vi "store constructor.vi"(11 "Store type":T1(array[ring])=[enum."AD_STORE_DISCRETE"]) -> (3 "Store ID":i32)   [LabVIEW 2021, in "libad4.lvlib"]
doc: "Helper to make setting the store type easier."
uses:
  <userlib>/libad4/libad4.lvlib
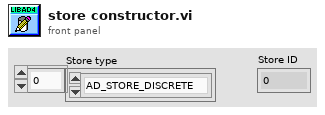
[diagram p1: front panel]
types:
  T1 = enum16{"AD_STORE_DISCRETE", "AD_STORE_AVERAGE", "AD_STORE_MIN", "AD_STORE_MAX", "AD_STORE_RMS"}[]
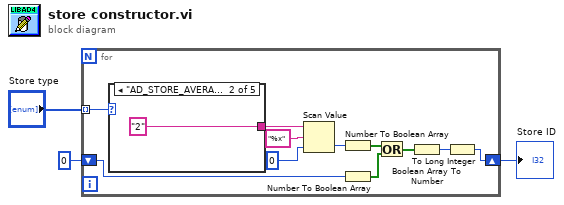
[diagram p0: block diagram]
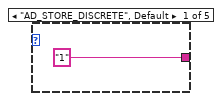
[diagram p2: hidden frame]
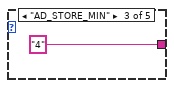
[diagram p3: hidden frame]
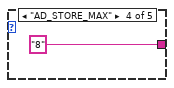
[diagram p4: hidden frame]
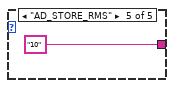
[diagram p5: hidden frame]
diagram:
  n1 = for {
    tunnel: "Store type" -> [w12] mode=indexing
    shift-right: [w6] -> w3
    shift-left: 0 -> [w5]
    n2 = case shown="\"AD_STORE_AVERAGE\"" w12 {
      tunnel: ["1" "2" "4" "8" "10"] -> w13
      frame "AD_STORE_DISCRETE", Default {
      }
      frame "AD_STORE_AVERAGE" {
      }
      frame "AD_STORE_MIN" {
      }
      frame "AD_STORE_MAX" {
      }
      frame "AD_STORE_RMS" {
      }
    }
    n3 = Scan Value(string=w13, format string="%x", default (0 dbl)=0) -> (value=w7:i32)  [unwired: 1 out]
    n4 = Number To Boolean Array(number=w7) -> (Boolean array=w9:bool[])
    n5 = Number To Boolean Array(number=w5) -> (Boolean array=w11:bool[])
    n6 = Or(x=w9, y=w11) -> (x .or. y?=w10:bool[])
    n7 = Boolean Array To Number(Boolean array=w10) -> (number=w8:i32)
    n8 = To Long Integer(number=w8) -> (32bit integer=w6:i32)
  }
  "Store ID" <- w3
